vi "GetStatusOnly.vi"(8 "error in (no error)":errorcluster, 11 "Value":string) -> (0 "error out":errorcluster, 2 "status":string, 3 "Found":bool)   [LabVIEW 2021]
uses:
  b3b0fdf2-cb34-410b-9075-fd36f45b70f0.vi
  <vilib>/JDP Science/JSONtext/Find Item.vi
  <vilib>/JDP Science/JSONtext/Next JSON Value.vi
  <vilib>/JDP Science/JSONtext/String Subset.vi
  <vilib>/JDP Science/JSONtext/Parsing/Advance past next JSON Value (inlined COPY).vi
  <vilib>/JDP Science/JSONtext/Parsing/Advance past whitespace.vi
  <vilib>/JDP Science/JSONtext/Parsing/Advance past String.vi
  <vilib>/JDP Science/JSONtext/Parsing/Advance past Number.vi
  <vilib>/JDP Science/JSONtext/Parsing/Advance past Line Ending.vi
  <vilib>/JDP Science/JSONtext/Parsing/Parse Full Path or Item Name.vi
  <vilib>/JDP Science/JSONtext/Parsing/Advance past Array.vi
  <vilib>/JDP Science/JSONtext/Parsing/Advance past Object.vi
  <vilib>/JDP Science/JSONtext/support/Error Cluster From Code.vi
  <vilib>/JDP Science/JSONtext/Offset/Find Item Locations by Path.vi
  <vilib>/JDP Science/JSONtext/JSON text to Variant.vi
  <vilib>/JDP Science/JSONtext/LVClass Serializer/JSONtext LVClass Serializer.lvclass
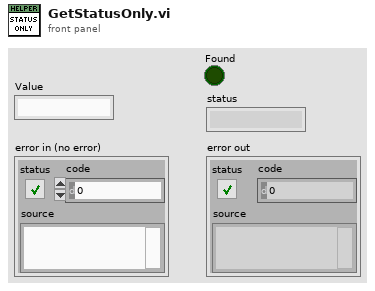
[diagram p1: front panel]
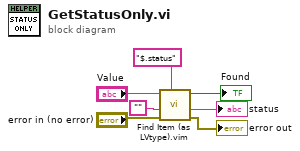
[diagram p0: block diagram]
diagram:
  n1 = call "Find Item (as LVtype).vim"("$Path or Item Name"="$.status", "error in (no error)"="error in (no error)", "Data Type and Default Value"="", "JSON"="Value") -> ("error out"=→"error out":errorcluster, "Data"=→"status":string, "Found"=→"Found":bool)  [unwired: 4 in, 1 out]
